vi "梦幻城堡C6~C20-WA解析.vi"(11 "读取缓冲区":string) -> (3 "Status":T1)   [LabVIEW 2016, in "环境动力监测库.lvlib" / "UPS库.lvlib"]
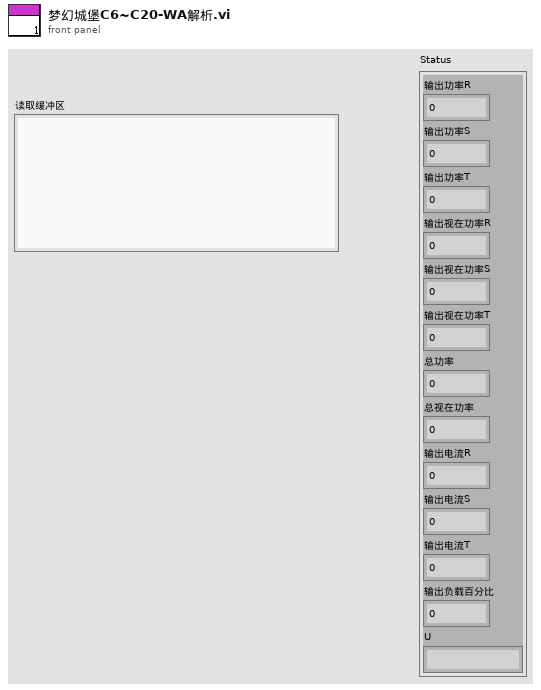
[diagram p1: front panel]
types:
  T1 = cluster{"输出功率R":dbl, "输出功率S":dbl, "输出功率T":dbl, "输出视在功率R":dbl, "输出视在功率S":dbl, "输出视在功率T":dbl, "总功率":dbl, "总视在功率":dbl, "输出电流R":dbl, "输出电流S":dbl, "输出电流T":dbl, "输出负载百分比":dbl, "U":string}
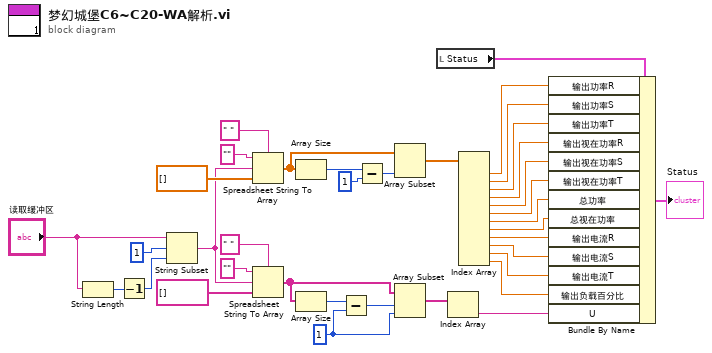
[diagram p0: block diagram]
diagram:
  w17 = 1 ("y")
  n1 = String Length(string="读取缓冲区") -> (length=w32:i32)
  n2 = Decrement(x=w32) -> (x-1=w31:i32)
  n3 = String Subset(string="读取缓冲区", offset (0)=1 ("偏移量(0)"), length (rest)=w31) -> (substring=w25:string)
  n4 = Spreadsheet String To Array(delimiter (Tab)=" " ("格式字符串"), format string="" ("格式字符串"), spreadsheet string=w25, array type (2D Dbl)=dbl[] []) -> (array=w24:dbl[])
  n5 = Spreadsheet String To Array(delimiter (Tab)=" " ("格式字符串"), format string="" ("格式字符串"), spreadsheet string=w25, array type (2D Dbl)=string[] []) -> (array=w19:string[])
  n6 = Array Size(array=w24) -> (size(s)=w23:i32)
  n7 = Array Size(array=w19) -> (size(s)=w20:i32)
  n8 = Subtract(x=w20, y=w17) -> (x-y=w18:i32)
  n9 = Subtract(x=w23, y=1) -> (x-y=w22:i32)
  n10 = Array Subset(array=w24, length=w22) -> (w16:dbl[])  [unwired: 1 in]
  n11 = Array Subset(array=w19, index=w18, length=w17) -> (w15:string[])
  n12 = local read "Status"() -> (w36:T1)
  n13 = Index Array(array=w15) -> (element=w1:string)  [unwired: 1 in]
  n14 = Index Array(array=w16) -> (element #1=w13:dbl, element #2=w12:dbl, element #3=w11:dbl, element #4=w10:dbl, element #5=w9:dbl, element #6=w8:dbl, element #7=w7:dbl, element #8=w6:dbl, element #9=w5:dbl, element #10=w4:dbl, element #11=w3:dbl, element #12=w2:dbl)  [unwired: 12 in]
  n15 = Bundle By Name(cluster=w36, "输出功率R"=w13, "输出功率S"=w12, "输出功率T"=w11, "输出视在功率R"=w10, "输出视在功率S"=w9, "输出视在功率T"=w8, "总功率"=w7, "总视在功率"=w6, "输出电流R"=w5, "输出电流S"=w4, "输出电流T"=w3, "输出负载百分比"=w2, "U"=w1) -> (→"Status":T1)
